vi "next.vi"(8 "error in (no error)":errorcluster, 11 "MissionQueue in":refnum<class "MissionQueue.lvclass">) -> (0 "error out":errorcluster, 1 "Valid?":bool, 2 "Mission.lvclass":refnum<class "Mission.lvclass">, 3 "MissionQueue out":refnum<class "MissionQueue.lvclass">)   [LabVIEW 2011]
uses:
  Mission/Mission.lvclass
  MissionQueue.lvclass
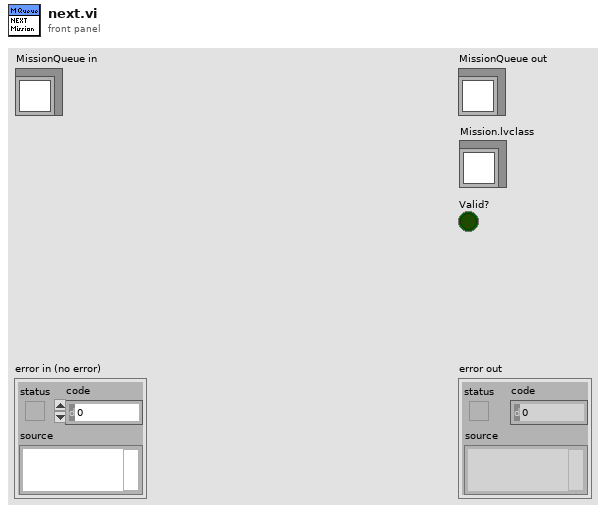
[diagram p1: front panel]
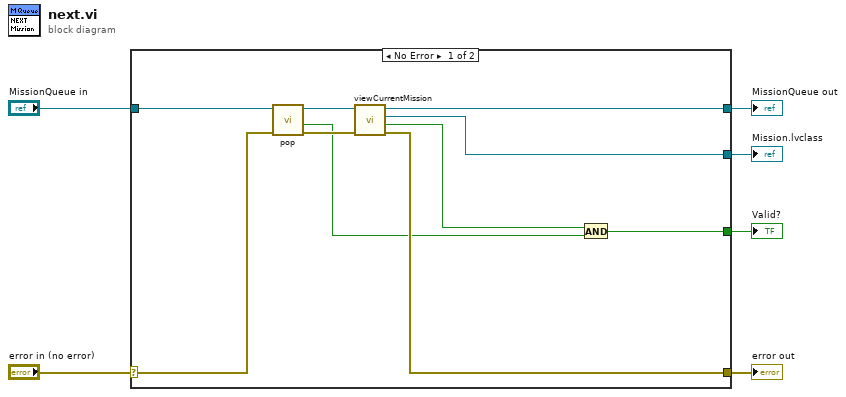
[diagram p0: block diagram]
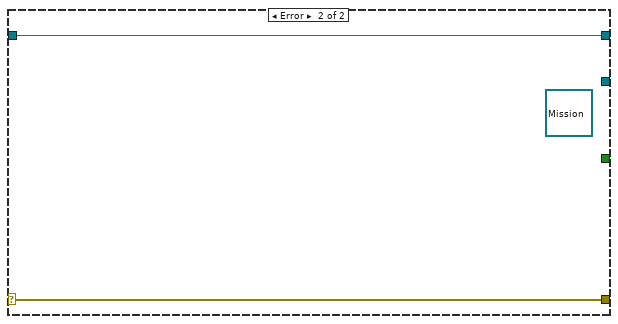
[diagram p2: hidden frame]
diagram:
  n1 = case shown="No Error" "error in (no error)" {
    selector: "error in (no error)" -> [w15 w18]
    tunnel: [w11 w18] -> w5
    tunnel: [w12 w17] -> w3
    tunnel: "MissionQueue in" -> [w16 w17]
    tunnel: [w10 _] -> w2
    tunnel: [w9 _] -> w1
    frame No Error {
      n2 = call "pop.vi"("error in (no error)"=w15, "MissionQueue in"=w16) -> ("error out"=w13:errorcluster, "Valid?"=w7:bool, "MissionQueue out"=w14:refnum<class "MissionQueue.lvclass">)  [unwired: 6 in, 1 out]
      n3 = call "viewCurrentMission.vi"("error in (no error)"=w13, "MissionQueue in"=w14) -> ("error out"=w11:errorcluster, "Valid?"=w8:bool, "Mission.lvclass"=w10:refnum<class "Mission.lvclass">, "MissionQueue out"=w12:refnum<class "MissionQueue.lvclass">)  [unwired: 6 in]
      n4 = And(x=w8, y=w7) -> (x .and. y?=w9:bool)
    }
    frame Error {
      (unwired) refnum<class "Mission.lvclass"> refnum ("Mission.lvclass")
    }
  }
  "error out" <- w5
  "MissionQueue out" <- w3
  "Valid?" <- w1
  "Mission.lvclass" <- w2
